vi "GDSError_ClearCustomError.vi"(5 "error in (no error)":errorcluster, 6 "ClearErrorCode":T1=enum."NoProductAccessGranted") -> (16 "Cleared?":bool, 19 "error out":errorcluster)   [LabVIEW 2020]
doc: "Use this VI to ignore errors with a certain code."
uses:
  <resource>/Framework/Providers/Open_GDS/SubVIs/GOOP_ErrorCodes.ctl
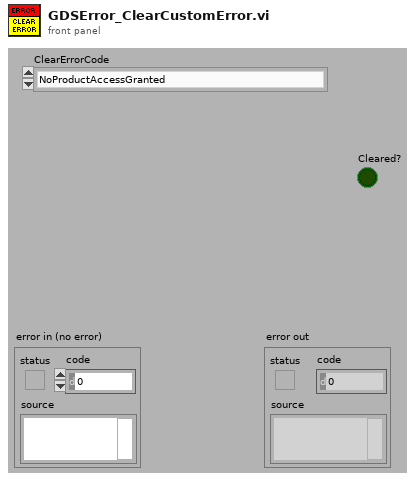
[diagram p1: front panel]
types:
  T1 = typedef "GOOP_ErrorCodes.ctl" = enum16{"LicenseFileMissing", "LicenseFileNotCorrect", "NoProductAccessGranted", "AgreementNoAccepted", "NoValidProviderFound", "LicenseExpired", "LanguageUndefined", "LanguageFileMissing", "LanguageFileChecksumError", "DublicateLanguageTranslation", "LanguageStringIDNotFound", "CommunityLimitReached", "ClassFileLocked", "ClassFileReadOnly", "ProjectNotValid"}
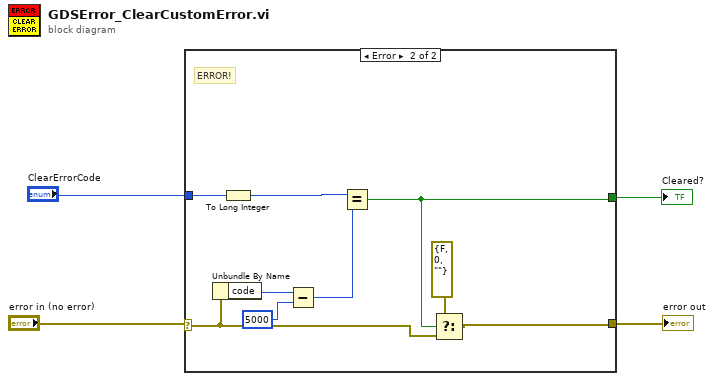
[diagram p0: block diagram]
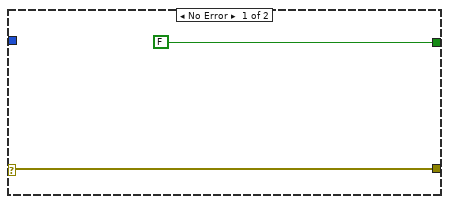
[diagram p2: hidden frame]
diagram:
  n1 = case shown="Error" "error in (no error)" {
    selector: "error in (no error)" -> [w5 w10]
    tunnel: [w5 w8] -> w4
    tunnel: [FALSE w9] -> w3
    tunnel: "ClearErrorCode" -> [_ w13]
    frame No Error {
    }
    frame Error {
      # "ERROR!"
      n2 = Unbundle By Name(w10) -> ("code"=w15:i32)
      n3 = To Long Integer(number=w13) -> (32bit integer=w12:i32)
      n4 = Subtract(x=w15, y=5000) -> (x-y=w11:i32)
      n5 = Equal?(x=w12, y=w11) -> (x = y?=w9:bool)
      n6 = Select(t=errorcluster {"status"=FALSE, "code"=0, "source"=""}, s=w9, f=w10) -> (s? t:f=w8:errorcluster)
    }
  }
  "error out" <- w4
  "Cleared?" <- w3
